vi "Initialize Async VIs.vi"(6 "VI in":refnum<vi>, 8 "error in (no error)":errorcluster, 10 "Async VI Parameters":variant[](array[variant]), 11 "Async VI Refs":refnum<vi>[](array[refnum])) -> (0 "error out":errorcluster, 3 "VI Ref In":refnum<vi>[](array[refnum]))   [LabVIEW 2013, in "Control Addon Engine.lvlib"]
uses:
  Control Addon Engine.lvlib
  Inline Async API/Controls/Parameters Cluster.ctl
  Inline Async API/Inline Async API.lvlib
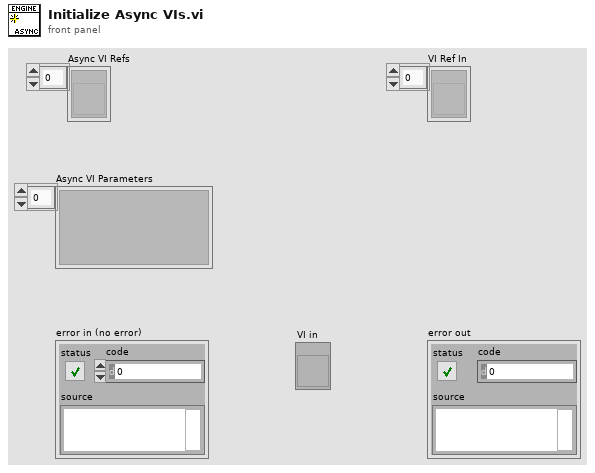
[diagram p1: front panel]
types:
  T1 = typedef "Control Addon Engine.lvlib/Inline Async API.lvlib/Parameters Cluster.ctl" = cluster{"Parameter Name":string, "Initial Settings":variant}
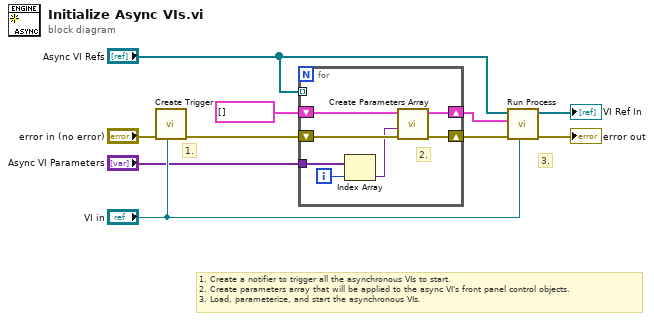
[diagram p0: block diagram]
diagram:
  # "1. Create a notifier to trigger all the asynchronous VIs to start.\n2. Create parameters array that will be applied to the async VI's front panel control objects.\n3. Load, parameterize, and start the asynchronous VIs."
  # "3."
  # "1."
  n1 = call "Create Trigger.vi"("This VI"="VI in", "error in (no error)"="error in (no error)") -> ("error out"=w6:errorcluster)  [unwired: 9 in]
  n2 = for {
    shift-right: [w17] -> w7
    shift-left: cluster{T1[]}[] [] ("Initial Parameters") -> [w14]
    shift-right: [w15] -> w5
    shift-left: w6 -> [w16]
    tunnel: "Async VI Refs" -> [_] mode=indexing
    tunnel: "Async VI Parameters" -> [w12]
    i -> [w13]
    # "2."
    n3 = Index Array(array=w12, index=w13) -> (element=w11:variant)
    n4 = call "Create Parameters Array.vi"("error in (no error)"=w16, "Initial Settings"=w11, "Initial Parameters"=w14) -> ("error out"=w15:errorcluster, "Initial Parameters"=w17:cluster{T1[]}[])  [unwired: 7 in]
  }
  n5 = call "Run Process.vi"("Parent VI"="VI in", "error in (no error)"=w5, "Initial Parameters"=w7, "VI Ref In"="Async VI Refs") -> ("error out"=→"error out":errorcluster, "VI Ref In"=→"VI Ref In":refnum<vi>[])  [unwired: 6 in]
